vi "DSF.Engine.Transfer Group.Set Debug Flags.vi"(10 "Debug Flags":refnum<class "DSF.Engine.Debug Flags.lvclass">, 11 "Transfer Group in":refnum<class "DSF.Engine.Transfer Group.lvclass">) -> (3 "Transfer Group out":refnum<class "DSF.Engine.Transfer Group.lvclass">)   [LabVIEW 2017, in "DSF.Engine.lvlib" / "DSF.Engine.Transfer Group.lvclass"]
uses:
  DSF.Engine.Transfer Group.lvclass
  Debug/DSF.Engine.Debug Flags.lvclass
  DSF.Engine.Transfer Group.lvclass/DSF.Engine.Transfer Group.ctl
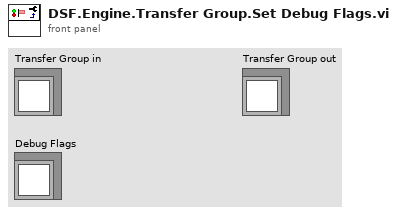
[diagram p1: front panel]
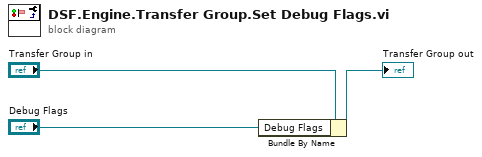
[diagram p0: block diagram]
diagram:
  n1 = Bundle By Name(cluster="Transfer Group in", "Debug Flags"="Debug Flags") -> (→"Transfer Group out":refnum<class "DSF.Engine.Transfer Group.lvclass">)
